vi "Init Build Spec.vi"(8 "error in (no error)":errorcluster, 11 "Builder in":refnum<class "Builder.lvclass">) -> (0 "error out":errorcluster, 2 "Added Version VI":bool, 3 "Builder out":refnum<class "Builder.lvclass">)   [LabVIEW 2019, in "Builder.lvclass"]
uses:
  Builder.lvclass
  TargetType.ctl
  Builder.lvclass/Builder.ctl
  d9ae1ceb-9950-4fe7-86c3-b3a01f98ca33.vi
  <vilib>/AppBuilder/AB_API/DPPL/NI_AB_API_DPPL.lvclass
  C:/Program Files (x86)/National Instruments/LabVIEW 2019/vi.lib/AppBuilder/AB_API/PPL/NI_AB_API_PPL.lvclass
  <vilib>/AppBuilder/AB_API/PPL/NI_AB_API_PPL.lvclass
  INI Parsing/PPL INI Parsing.lvlib
  C:/Program Files (x86)/National Instruments/LabVIEW 2019/vi.lib/AppBuilder/AB_API/Targetfile/NI_AB_API_Targetfile.lvclass
  C:/Program Files (x86)/National Instruments/LabVIEW 2019/vi.lib/AppBuilder/AB_API/Build/NI_AB_API_Build.lvclass
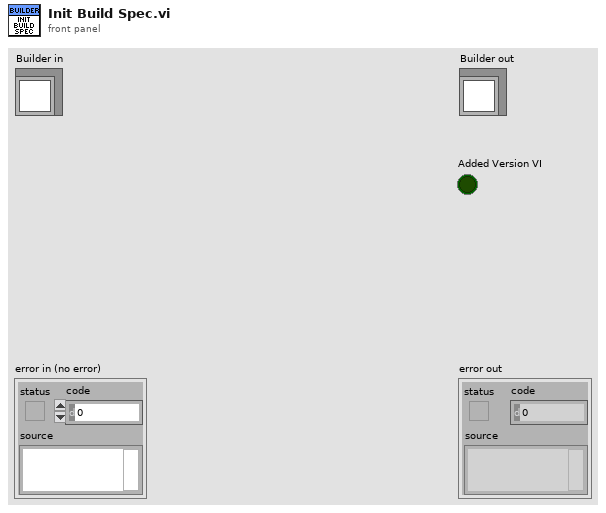
[diagram p1: front panel]
types:
  T1 = typedef "TargetType.ctl" = enum16{"Windows", "cRIO-9045"}
  T2 = cluster{"Major":i32, "Minor":i32, "Patch":i32, "Build":i32}
  T3 = typedef "PPL INI Parsing.lvlib/Build Configuration.ctl" = cluster{"SV Pairs":string[][], "Description":string}
  T4 = typedef "Builder.lvclass/Builder Configuration.ctl" = cluster{"Company":string, "CopyrightHolder":string, "InternalPrefix":string}
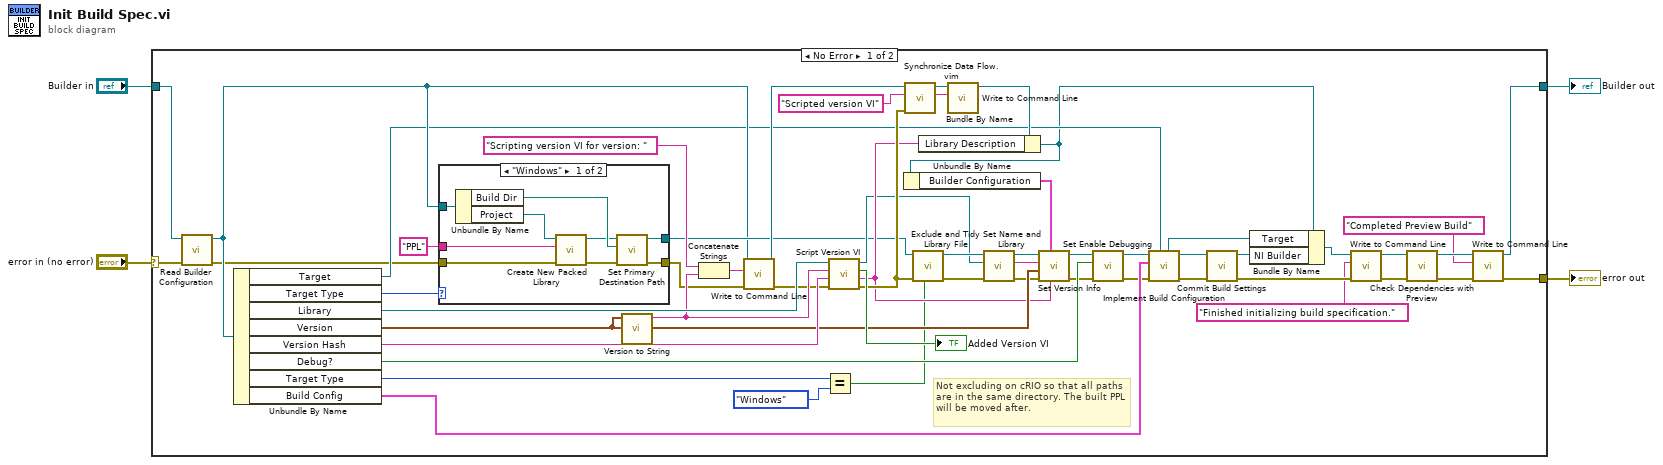
[diagram p0: block diagram]
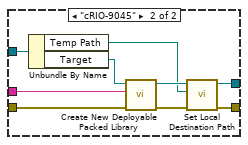
[diagram p2: hidden frame]
diagram:
  n1 = case shown="No Error" "error in (no error)" {
    selector: "error in (no error)" -> [w11 w79]
    tunnel: [w21 w79] -> w3
    tunnel: [w19 w78] -> w1
    tunnel: "Builder in" -> [w9 w78]
    frame No Error {
      # "Not excluding on cRIO so that all paths are in the same directory. The built PPL will be moved after."
      n2 = call "Read Builder Configuration.vi"("error in (no error)"=w11, "Builder in"=w9) -> ("error out"=w7:errorcluster, "Builder out"=w10:refnum<class "Builder.lvclass">)  [unwired: 8 in]
      n3 = Unbundle By Name(w10) -> ("Target"=w8:refnum<vi>, "Target Type"=w49:T1, "Library"=w50:refnum<vi>, "Version"=w55:T2, "Version Hash"=w56:string, "Debug?"=w51:bool, "Target Type"=w48:T1, "Build Config"=w42:T3)
      n4 = case shown="\"Windows\"" w49 {
        tunnel: w7 -> [w66 w77]
        tunnel: "PPL" ("Build specification name") -> [w67 w76]
        tunnel: [w64 w74] -> w17
        tunnel: [w62 w72] -> w24
        tunnel: w10 -> [w61 w71]
        frame "Windows" {
          n5 = Unbundle By Name(w61) -> ("Build Dir"=w68:path, "Project"=w60:refnum<vi>)
          n6 = call <vilib>:"Create New Packed Library.vi"("error in (no error)"=w66, "Build specification name"=w67, "Project Refnum"=w60) -> ("error out"=w63:errorcluster, "PPL out"=w65:refnum<class "NI_AB_API_PPL.lvclass">)  [unwired: 7 in]
          n7 = call-dynamic "Set Primary Destination Path.vi"("error in (no error)"=w63, "Destination path"=w68, "Build in"=w65) -> ("error out"=w62:errorcluster, "Build out"=w64:refnum<class "NI_AB_API_PPL.lvclass">)  [unwired: 7 in]
        }
        frame "cRIO-9045" {
          n8 = Unbundle By Name(w71) -> ("Temp Path"=w70:path, "Target"=w69:refnum<vi>)
          n9 = call <vilib>:"Create New Deployable Packed Library.vi"("error in (no error)"=w77, "Build specification name"=w76, "TargetItem Refnum"=w69) -> ("error out"=w73:errorcluster, "PPL out"=w75:refnum<class "NI_AB_API_DPPL.lvclass">)  [unwired: 7 in]
          n10 = call <vilib>:"Set Local Destination Path.vi"("error in (no error)"=w73, "Local destination path"=w70, "NI_AB_API_DPPL in"=w75) -> ("error out"=w72:errorcluster, "NI_AB_API_DPPL out"=w74:refnum<class "NI_AB_API_DPPL.lvclass">)  [unwired: 7 in]
        }
      }
      n11 = call "Version to String.vi"("Version"=w55) -> ("String"=w26:string)  [unwired: 10 in]
      n12 = Concatenate Strings("Scripting version VI for version: " ("string"), w26) -> (w25:string)
      n13 = call "Write to Command Line.vi"("error in (no error)"=w24, "Message"=w25, "Builder in"=w10) -> ("error out"=w23:errorcluster, "Builder out"=w59:refnum<class "Builder.lvclass">)  [unwired: 7 in]
      n14 = Equal?(x=w48, y=TargetType."Windows") -> (x = y?=w28:bool)
      n15 = call "Script Version VI.vi"("error in (no error)"=w23, "Commit Reference"=w56, "Version String"=w26, "Library Refnum"=w50) -> ("error out"=w57:errorcluster, "Library Description"=w30:string, "Added Version VI"=→"Added Version VI":bool, "Library Refnum out"=w27:refnum<vi>)  [unwired: 4 in]
      n16 = call "Synchronize Data Flow.vim"("input 4"=w57, "input 2"="Scripted version VI" ("Message"), "input 1"=w59) -> ("output 2"=w13:string, "output 1"=w14:refnum<class "Builder.lvclass">)  [unwired: 1 in, 2 out]
      n17 = call "Exclude and Tidy Library File.vi"("Exclude dependent packed libraries (T)"=w28, "error in (no error)"=w57, "NI_AB_API_PPL in"=w17) -> ("error out"=w33:errorcluster, "NI_AB_API_PPL out"=w35:refnum<class "NI_AB_API_PPL.lvclass">)  [unwired: 7 in]
      n18 = call "Write to Command Line.vi"("Message"=w13, "Builder in"=w14) -> ("Builder out"=w22:refnum<class "Builder.lvclass">)  [unwired: 8 in, 1 out]
      n19 = Bundle By Name(cluster=w22, "Library Description"=w30) -> (w6:refnum<class "Builder.lvclass">)
      n20 = Unbundle By Name(w6) -> ("Builder Configuration"=w5:T4)
      n21 = call "Set Name and Library.vi"("error in (no error)"=w33, "Top-Level Library Ref"=w27, "NI_AB_API_PPL in"=w35) -> ("error out"=w16:errorcluster, "PPL Name"=w36:string, "NI_AB_API_PPL out"=w37:refnum<class "NI_AB_API_PPL.lvclass">)  [unwired: 6 in]
      n22 = call "Set Version Info.vi"("Description"=w30, "Builder Configuration"=w5, "error in (no error)"=w16, "Build Spec Version"=w55, "Name"=w36, "NI_AB_API_PPL in"=w37) -> ("error out"=w12:errorcluster, "NI_AB_API_PPL out"=w34:refnum<class "NI_AB_API_PPL.lvclass">)  [unwired: 4 in]
      n23 = call-dynamic "Set Enable Debugging.vi"("error in (no error)"=w12, "Enable debugging (false)"=w51, "PPL in"=w34) -> ("error out"=w32:errorcluster, "PPL out"=w46:refnum<class "NI_AB_API_PPL.lvclass">)  [unwired: 7 in]
      n24 = call "Implement Build Configuration.vi"("Target in"=w8, "error in (no error)"=w32, "Build Config"=w42, "PPL in"=w46) -> ("error out"=w45:errorcluster, "PPL out"=w47:refnum<class "NI_AB_API_PPL.lvclass">, "Target out"=w41:refnum<vi>)  [unwired: 5 in]
      n25 = call-dynamic "Commit Build Settings.vi"("error in (no error)"=w45, "PPL in"=w47) -> ("error out"=w44:errorcluster, "PPL out"=w43:refnum<class "NI_AB_API_PPL.lvclass">)  [unwired: 8 in]
      n26 = Bundle By Name(cluster=w6, "Target"=w41, "NI Builder"=w43) -> (w39:refnum<class "Builder.lvclass">)
      n27 = call "Write to Command Line.vi"("error in (no error)"=w44, "Message"="Finished initializing build specification.", "Builder in"=w39) -> ("error out"=w40:errorcluster, "Builder out"=w29:refnum<class "Builder.lvclass">)  [unwired: 7 in]
      n28 = call "Check Dependencies with Preview.vi"("error in (no error)"=w40, "Builder in"=w29) -> ("error out"=w31:errorcluster, "Builder out"=w20:refnum<class "Builder.lvclass">)  [unwired: 8 in]
      n29 = call "Write to Command Line.vi"("error in (no error)"=w31, "Message"="Completed Preview Build", "Builder in"=w20) -> ("error out"=w21:errorcluster, "Builder out"=w19:refnum<class "Builder.lvclass">)  [unwired: 7 in]
    }
    frame Error {
    }
  }
  "error out" <- w3
  "Builder out" <- w1
